vi "Write String Configuration.vi"(8 "error in (no error)":errorcluster, 9 "Value":string, 10 "Name":string, 11 "IniFileSection in":refnum<class "IniFileSection.lvclass">) -> (0 "error out":errorcluster, 3 "IniFileSection out":refnum<class "IniFileSection.lvclass">)   [LabVIEW 2020, in "IniFileSection.lvclass"]
uses:
  <vilib>/gpm_packages/@cs/Configuration/Source/IniFileSection/IniFileSection.lvclass
  <vilib>/gpm_packages/@cs/Configuration/Source/IniFileSection/IniFileSection.lvclass/IniFileSection.ctl
  <vilib>/Utility/config.llb/Write Key (String).vi
  <vilib>/Utility/config.llb/NI_LVConfig.lvlib
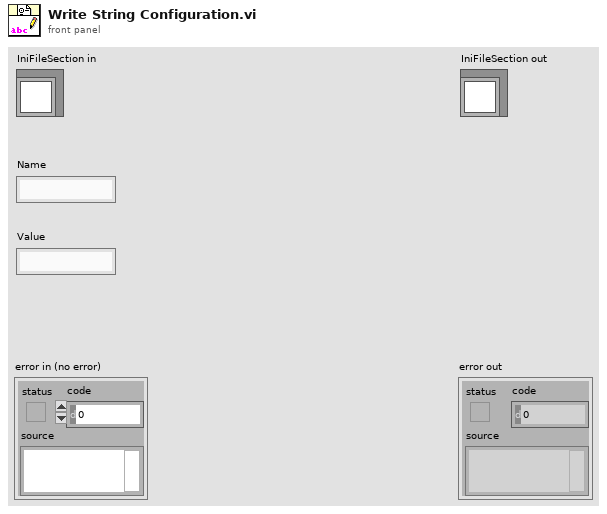
[diagram p1: front panel]
types:
  T1 = typedef "NI_LVConfig.lvlib/Config Data RefNum.ctl" = refnum<k1>
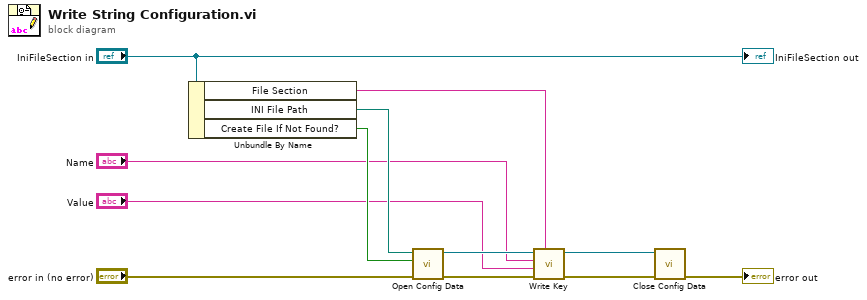
[diagram p0: block diagram]
diagram:
  n1 = Unbundle By Name("IniFileSection in") -> ("File Section"=w7:string, "INI File Path"=w8:path, "Create File If Not Found?"=w6:bool)
  n2 = call <vilib>:"Open Config Data.vi"("error in (no error)"="error in (no error)", "create file if necessary (T)"=w6, "configuration file path"=w8) -> ("error out"=w12:errorcluster, "refnum"=w10:T1)  [unwired: 6 in, 1 out]
  n3 = call-poly <vilib>:"Write Key.vi"("section"=w7, "error in (no error)"=w12, "value"="Value", "key"="Name", "refnum"=w10) -> ("error out"=w11:errorcluster, "refnum out"=w9:T1)  [unwired: 4 in, 1 out]
  n4 = call <vilib>:"Close Config Data.vi"("error in (no error)"=w11, "refnum"=w9) -> ("error out"=→"error out":errorcluster)  [unwired: 8 in, 1 out]
  "IniFileSection out" <- "IniFileSection in"
